vi "Read Manager.Text Configuration.vi"(11 "ConfigManager.Text in":refnum<class "ConfigManager.Text.lvclass">) -> (2 "Manager.Text Configuration":T1, 3 "ConfigManager.Text out":refnum<class "ConfigManager.Text.lvclass">)   [LabVIEW 2013, in "CfgManager.Text.lvlib" / "ConfigManager.Text.lvclass"]
uses:
  ConfigManager.Text.lvclass
  Configuration -- Cluster.ctl
  FileHeader/FileHeader.lvclass
  FileSignature/FileSignature.lvclass
  <vilib>/LabVIEW Open Source Project/Unicity/Delimiter/Delimiter.lvclass
  ConfigManager.Text.lvclass/ConfigManager.Text.ctl
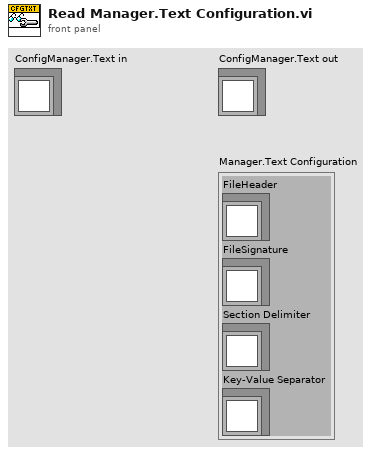
[diagram p1: front panel]
types:
  T1 = typedef "CfgManager.Text.lvlib/ConfigManager.Text.lvclass/Configuration -- Cluster.ctl" = cluster{"FileHeader":refnum<class "FileHeader.lvclass">, "FileSignature":refnum<class "FileSignature.lvclass">, "Section Delimiter":refnum<class "Delimiter.lvclass">, "Key-Value Separator":refnum<class "Delimiter.lvclass">}
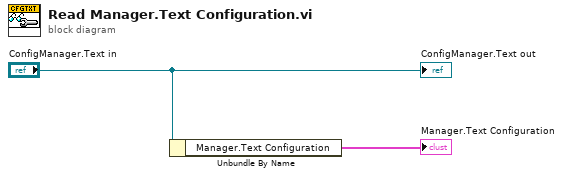
[diagram p0: block diagram]
diagram:
  n1 = Unbundle By Name("ConfigManager.Text in") -> ("Manager.Text Configuration"=→"Manager.Text Configuration":T1)
  "ConfigManager.Text out" <- "ConfigManager.Text in"
